vi "PendRealtime_IP5.vi"() -> ()   [LabVIEW 2012]
doc: "This VI was generated automatically using the FPGA Wizard. You can modify the VI normally."
uses:
  <vilib>/Platform/TimedLoop/XDataNode/timing_clust.ctl
  <vilib>/Platform/TimedLoop/XDataNode/nitl_modes.ctl
  <vilib>/Platform/TimedLoop/XDataNode/wakeup.ctl
  <vilib>/FPGAPlugInAG/sbRIO-9632/niLvFpga_Open_sbRIO-9632.vi
  <vilib>/rvi/interface/common/dynamic/niFpgaDynamicAddResources.vi
  <vilib>/FPGAPlugInAG/Dynamic/niLvFpga_Reset_Dynamic.vi
  <vilib>/FPGAPlugInAG/Dynamic/niLvFpga_Run_Dynamic.vi
  <vilib>/Utility/error.llb/Error Cluster From Error Code.vi
  <vilib>/rvi/errors/niLvFpgaAdjustHostInterfaceError.vi
  <vilib>/FPGAPlugInAG/Dynamic/niLvFpga_Close_Dynamic.vi
  <vilib>/rvi/interface/nirviOpenFPGA/nirviOpenFPGA.xnode
  FPGA Bitfiles/PPDControlLab3_FPGA_IP5.lvbitx
  <vilib>/rvi/interface/nirviMethod/nirviMethod.xnode
  <vilib>/Platform/TimedLoop/XDataNode/XDataNode.xnode
  <vilib>/rvi/interface/nirviReadWriteControl/nirviReadWriteControl.xnode
  <vilib>/rvi/interface/nirviCloseFPGA/nirviCloseFPGA.xnode
  SysIDRealtime.lvlib
  <vilib>/rvi/interface/Simulation/niFpgaSimulationCallBeginRW.vi
  <vilib>/Platform/TimedLoop/XDataNode/XDNodeRunTimeDep.lvlib
  NiFpgaLv.dll
panel:
  in  "K3":dbl=32.996501911713274
  in  "K4":dbl=3.4016071395471763
  in  "K1":dbl=-0.3249
  in  "K2":dbl=-1.0317
  out "Enabled":bool=TRUE
  in  "Enable Control":bool=TRUE
  out "Control":fxp<+/-,20,5>
  in  "K4'":dbl=0.002609032676032684
  in  "K3'":dbl=0.0461262
  in  "K2'":dbl=1.0317e-06
  in  "K1'":dbl=3.249e-07
  out "Pendulum Position":i32=-6910
  out "Pendulum Response":dynamicdata(graph)=[{"t0"=timestamp(0 s since 1904-01-01), "dt"=1.0, "Y"=array[8192 elements]}, {"t0"=timestamp(0 s since 1904-01-01), "dt"=1.0, "Y"=array[53587 elements]}]
  out "Ratio":fxp<+/-,32,7>
  in  "Gain":fxp<+/-,32,7>=0.006999999284744263
  in  "Radio Buttons":enum32{"Radio Selection 1", "Radio Selection 2"}(radio)
  in  "OK Button":bool
  out "Step Response":dynamicdata(graph)=[{"t0"=timestamp(0 s since 1904-01-01), "dt"=1.0, "Y"=array[8192 elements]}, {"t0"=timestamp(0 s since 1904-01-01), "dt"=1.0, "Y"=array[8192 elements]}, {"t0"=timestamp(0 s since 1904-01-01), "dt"=1.0, "Y"=array[8192 elements]}]
  in  "samples":i32=8192
  in  "Reference":i32=100000
  in  "Quad Reset":bool=TRUE
  in  "DGain":fxp<+/-,32,7>
  in  "PGain":fxp<+/-,32,7>=-0.006999999284744263
  out "Amp In":dbl[](graph)
  out "Amp Cpmmand":fxp<+/-,20,5>=-16.0
  out "Iteration Duration":i64=1663
  out "Position":i32[](graph)
  in  "Control Rate (ticks)":u32=10000
  in  "Period (us)":i64=1000
  out "Finished Late? [i-1]":bool=TRUE
  out "quad saved (Port0/DIO0,Port0/DIO1)":cluster{"Position":i32, "Index Count":u16}={"Position"=-185790, "Index Count"=8041}
  out "quad pos (Port0/DIO0,Port0/DIO1)":i32=-185792
  out "Late? Latched":bool=TRUE
  in  "Local Stop 0":bool
  in  "Start 0":bool
  in  "Loop Rate (Hz)":dbl=100000.0
  out "Calculated Rate (Hz)":dbl=100000.0
  out "error out":errorcluster
  in  "Global Stop":bool
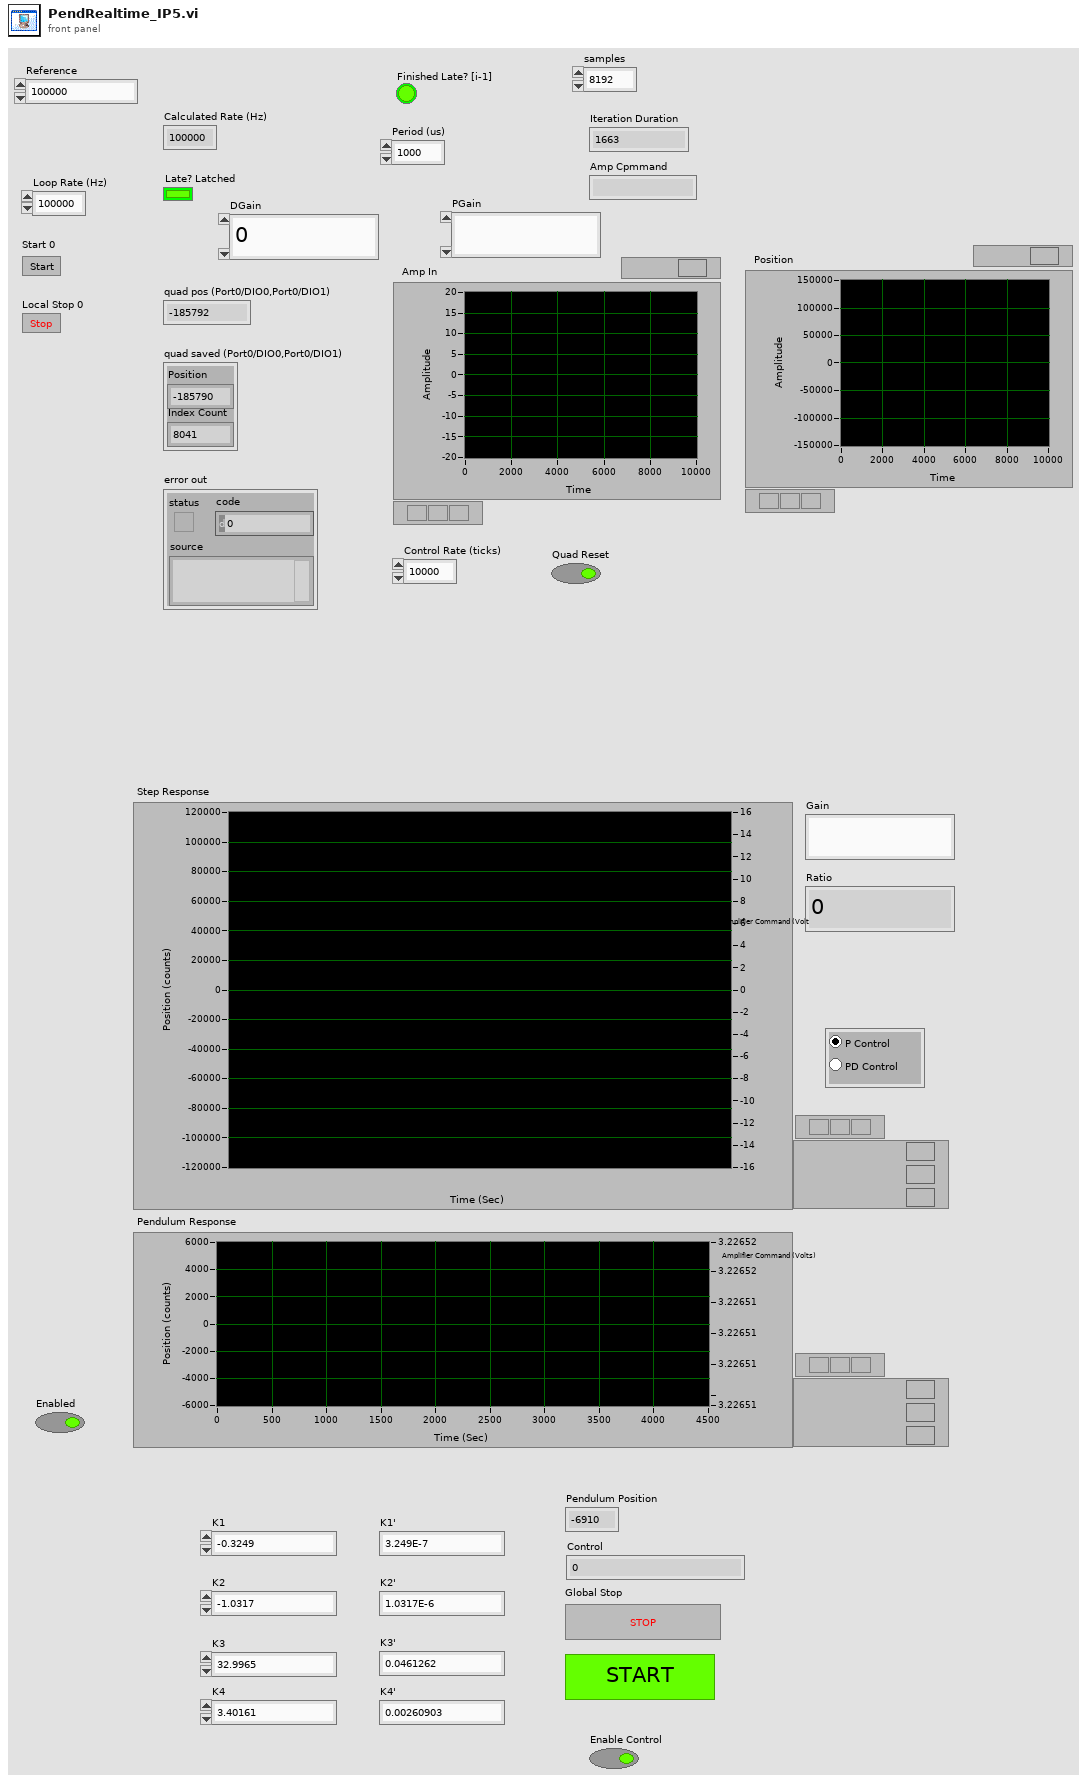
[diagram p1: front panel]
types:
  T1 = typedef "XDNodeRunTimeDep.lvlib/timing_clust.ctl" = cluster{"Expected End [f-1]":u64, "Actual End [f-1]":u64, "Finished Late? [f-1]":bool, "Expected End [i-1]":u64, "Actual End [i-1]":u64, "Finished Late? [i-1]":bool, "Expected Start [i]":u64, "Actual Start [i]":u64, "Expected Start [f]":u64, "Actual Start [f]":u64, "Source Name":string, "Structure Name":string, "Period":i64, "Deadline":i64, "Offset":i64, "Start":i64, "Priority":i32, "Timeout":i32, "Mode":T2, "Wakeup Reason":T3, "Error":errorcluster, "Source Type":string, "Secondary Source Type":string, "Global End Time":u64, "Global Start Time":u64, "Frame Duration":u64, "Iteration Duration":u64, "Assigned CPU":i32, "I/O Scan Engine Mode":u32}
  T2 = typedef "XDNodeRunTimeDep.lvlib/nitl_modes.ctl" = enum32{"No Change", "Process missed periods, maintain original phase", "Discard missed periods, maintain original phase", "Process missed periods, ignore original phase", "Discard missed periods, ignore original phase"}
  T3 = typedef "XDNodeRunTimeDep.lvlib/wakeup.ctl" = enum32{"Normal", "Aborted", "Asynchronous wakeup", "Timing source error", "Timed loop error", "Timeout"}
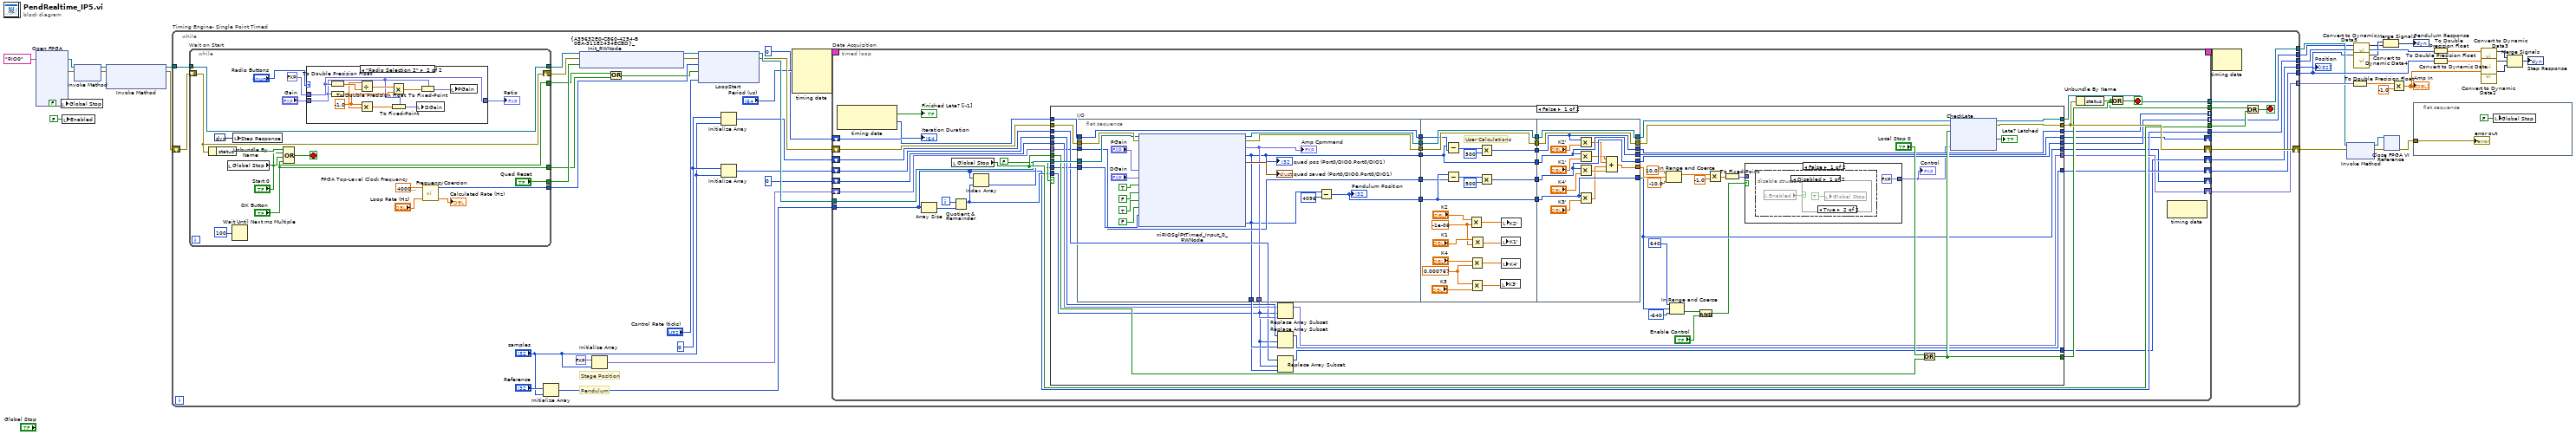
[diagram p0: block diagram]
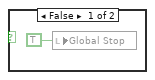
[diagram p2: hidden frame]
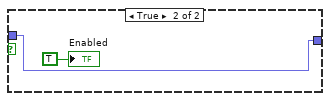
[diagram p4: hidden frame]
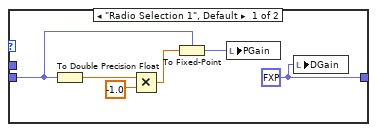
[diagram p6: hidden frame]
diagram:
  n1 = xnode ("Open FPGA")("resource name"=tag "RIO0") -> ("FPGA VI Reference Out"=w29:refnum<k20>, "error out"=w30:errorcluster)  [unwired: 1 in]
  n2 = local write "Global Stop"(FALSE ("Global Stop")) -> ()
  n3 = local write "Enabled"(FALSE ("Enabled")) -> ()
  n4 = xnode ("Invoke Method")("FPGA VI Reference In"=w29, "error in"=w30) -> ("FPGA VI Reference Out"=w12:refnum<k20>, "error out"=w11:errorcluster)
  n5 = xnode ("Invoke Method")("FPGA VI Reference In"=w12, "error in"=w11) -> ("FPGA VI Reference Out"=w17:refnum<k20>, "error out"=w31:errorcluster)  [unwired: 1 in]
  n6 = while "Timing Engine- Single Point Timed" {
    tunnel: w17 -> [w65]
    shift-right: [w64] -> w15
    shift-left: w31 -> [w68]
    tunnel: [w47] -> w23
    tunnel: [w48] -> w27
    tunnel: [w43] -> w21
    tunnel: [w39] -> w16
    tunnel: [w35] -> w7
    tunnel: [w32] -> w5
    stop <- w59 stop-if-true
    w38 = 0 ("quad pos (Port0/DIO0,Port0/DIO1)")
    # "Pendulum"
    # "Stage Position"
    n7 = while "Wait on Start" {
      tunnel: w65 -> [w240]
      tunnel: [w240] -> w63
      tunnel: [w232] -> w56
      tunnel: ["Start 0"] -> w42
      shift-right: [w234] -> w62
      shift-left: w68 -> [w234]
      tunnel: ["Quad Reset"] -> w46
      tunnel: ["OK Button"] -> w41
      stop <- w241 stop-if-true
      w235 = 40000000.0  # FPGA Top-Level Clock Frequency
      n8 = Unbundle By Name(w234) -> ("status"=w233:bool)
      n9 = local read "Global Stop"() -> (w238:bool)
      n10 = Wait Until Next ms Multiple(millisecond multiple=u32 100) -> ()  [unwired: 1 out]
      n11 = local write "Step Response"(dynamicdata [] ("Step Response")) -> ()
      n12 = Compound Arithmetic op=OR(w233, "Start 0", w238, "OK Button") -> (w241:bool)
      n13 = case shown="\"Radio Selection 2\"" "Radio Buttons" {
        tunnel: "Gain" -> [w243 w249]
        tunnel: fxp<+/-,32,7> 40.0 ("Ratio") -> [_ w254]
        tunnel: [w247 w254] -> w225
        frame "Radio Selection 1", Default {
          w247 = fxp<+/-,32,7> 0.0 ("DGain")
          n14 = To Double Precision Float(number=w243) -> (double precision float=w246:dbl)
          n15 = Multiply(x=w246, y=-1.0) -> (x*y=w244:dbl)
          n16 = To Fixed-Point(fixed-point type=w243, number=w244) -> (fixed-point=w242:fxp<+/-,32,7>)
          n17 = local write "PGain"(w242) -> ()
          n18 = local write "DGain"(w247) -> ()
        }
        frame "Radio Selection 2" {
          w252 = -1.0 ("y")
          n19 = To Double Precision Float(number=w254) -> (double precision float=w257:dbl)
          n20 = To Double Precision Float(number=w249) -> (double precision float=w251:dbl)
          n21 = Divide(x=w251, y=w257) -> (x/y=w256:dbl)
          n22 = Multiply(x=w252, y=w251) -> (x*y=w250:dbl)
          n23 = Multiply(x=w256, y=w252) -> (x*y=w253:dbl)
          n24 = To Fixed-Point(fixed-point type=w249, number=w250) -> (fixed-point=w248:fxp<+/-,32,7>)
          n25 = local write "DGain"(w248) -> ()
          n26 = To Fixed-Point(fixed-point type=w249, number=w253) -> (fixed-point=w255:fxp<+/-,32,7>)
          n27 = local write "PGain"(w255) -> ()
        }
      }
      "Ratio" <- w225
      n28 = call "FrequencyCoercion.vi"("Loop Rate (Hz)"="Loop Rate (Hz)", "FPGA Top-Level Clock Frequency"=w235) -> ("Actual Rate (Hz)"=→"Calculated Rate (Hz)":dbl, "FPGA Ticks"=w232:u32)  [unwired: 2 in]
    }
    n29 = Initialize Array("Reference", "samples") -> (w44:i32[])
    n30 = xnode ("{A39632E0-C860-4254-B0EA-311E2434ECBD}_Init_RWNode")("FPGA VI Reference In"=w63, "error in"=w62, "quad reset (Port0/DIO0,Port0/DIO1)"=w46) -> ("FPGA VI Reference Out"=w57:refnum<k20>, "error out"=w61:errorcluster)
    n31 = Initialize Array(fxp<+/-,20,5> 0.0 ("Amp Cpmmand"), "samples") -> (w49:fxp<+/-,20,5>[])
    n32 = Or(x=w42, y=w41) -> (x .or. y?=w40:bool)
    n33 = xnode ("LoopStart")("FPGA VI Reference In"=w57, "error in"=w61, "Loop Rate (Ticks)"=w56, "Start 0"=w40, "Control Rate (ticks)"="Control Rate (ticks)") -> ("FPGA VI Reference Out"=w67:refnum<k20>, "error out"=w66:errorcluster)
    n34 = Initialize Array(w38, "samples") -> (w36:i32[])
    n35 = Initialize Array(w38, "samples") -> (w51:i32[])
    n36 = node-c288("Period (us)") -> (w55:T1)  [unwired: 3 in]
    n37 = timed-loop "Data Acquisition" {
      tunnel: w67 -> [w91]
      tunnel: [w93] -> w60
      tunnel: [w92] -> w58
      shift-right: [w96] -> w64
      shift-left: w66 -> [w90]
      timing: w55 -> [_]
      timing-out: [_] -> w54
      tunnel: w44 -> [w78]
      shift-right: [w79] -> w48
      shift-left: w49 -> [w81]
      shift-right: [w80] -> w47
      shift-left: w51 -> [w83]
      tunnel: [w78] -> w43
      tunnel: [w77] -> w39
      shift-right: [w75] -> w35
      shift-left: w36 -> [w76]
      shift-right: [w72] -> _
      shift-left: 0 ("Pendulum Position") -> [w74]
      shift-right: [w70] -> _
      shift-left: 0 ("Stage Position") -> [w73]
      tunnel: [w69] -> _ mode=indexing
      tunnel: [w71] -> w32 mode=indexing
      i -> [w87]
      stop <- w94 stop-if-true
      n38 = node-c288() -> (→"Finished Late? [i-1]":bool, →"Iteration Duration":i64)  [unwired: 1 in]
      n39 = Array Size(array=w78) -> (size(s)=w85:i32)
      n40 = local read "Global Stop"() -> (w93:bool)
      n41 = Quotient & Remainder(x=w87, y=w85) -> (x-y*floor(x/y)=w84:i32)  [unwired: 1 out]
      n42 = Index Array(array=w78, index=w84) -> (element=w86:i32)
      n43 = case "Timeout" shown="False" FALSE {
        tunnel: w91 -> [w147 w217]
        tunnel: w90 -> [w146 w219]
        tunnel: [w140 w219] -> w96
        tunnel: [w142 w218] -> w95
        tunnel: w93 -> [w143 w218]
        tunnel: w86 -> [w133 _]
        tunnel: w84 -> [w130 _]
        tunnel: w83 -> [w138 _]
        tunnel: [w137 _] -> w80
        tunnel: w81 -> [w136 _]
        tunnel: [w134 _] -> w79
        tunnel: [w132 w217] -> w77
        tunnel: w76 -> [w131 _]
        tunnel: [w128 _] -> w75
        tunnel: [w110 w215] -> w72
        tunnel: [w125 w216] -> w70
        tunnel: w74 -> [w121 w215]
        tunnel: w73 -> [w119 w216]
        tunnel: [w118 _] -> w71
        tunnel: [w116 _] -> w69
        frame False {
          n44 = flat-sequence "I/O" {
            tunnel: w147 -> [w175]
            tunnel: w146 -> [w177]
            tunnel: [w176] -> w152
            tunnel: [w174] -> w149
            tunnel: [w162] -> w139
            tunnel: [w172] -> w135
            tunnel: w133 -> [w165]
            tunnel: [w161] -> w129
            tunnel: [w159] -> w126
            tunnel: [w162] -> w123
            tunnel: [w164] -> w122
            tunnel: w121 -> [w164]
            tunnel: [w163] -> w120
            tunnel: w119 -> [w163]
            tunnel: [w199] -> w151
            tunnel: w152 -> [w198]
            tunnel: w149 -> [w199]
            tunnel: [w198] -> w150
            tunnel: [w197] -> w127
            tunnel: w126 -> [w197]
            tunnel: [w194] -> w124
            tunnel: w123 -> [w194]
            tunnel: w122 -> [w196]
            tunnel: w120 -> [w195]
            tunnel: [w191] -> w117
            tunnel: [w188] -> w115
            tunnel: [w213] -> w145
            tunnel: [w214] -> w148
            tunnel: w151 -> [w214]
            tunnel: w150 -> [w213]
            tunnel: [w207] -> w110
            tunnel: w127 -> [w207]
            tunnel: [w205] -> w125
            tunnel: w124 -> [w205]
            tunnel: [w208] -> w118
            tunnel: w117 -> [w208]
            tunnel: [w206] -> w116
            tunnel: w115 -> [w206]
            tunnel: [w200] -> w114
            frame #0 {
              n45 = xnode ("niRIOSglPtTimed_Input_0_RWNode")("FPGA VI Reference In"=w175, "error in"=w177, "PGain"="PGain", "DGain"="DGain", "Amp Enable"=TRUE, "Amp Reset"=FALSE, "Brake"=TRUE, "quad reset (Port0/DIO0,Port0/DIO1)"=FALSE, "Reference"=w165) -> ("FPGA VI Reference Out"=w174:refnum<k20>, "error out"=w176:errorcluster, "Amp Cpmmand"=w172:fxp<+/-,20,5>, "Stage Position"=w162:i32, "quad saved (Port0/DIO0,Port0/DIO1)"=→"quad saved (Port0/DIO0,Port0/DIO1)":cluster{"Position":i32, "Index Count":u16}, "Pendulum Position"=w161:i32)
              "quad pos (Port0/DIO0,Port0/DIO1)" <- w162
              "Amp Cpmmand" <- w172
              n46 = Subtract(x=w161, y=4096 ("x")) -> (x-y=w159:i32)
              "Pendulum Position" <- w159
            }
            frame #1 {
              w179 = 0.000767 ("y")
              w184 = -1e-06 ("y")
              # "User Calculations"
              n47 = Subtract(x=w194, y=w195) -> (x-y=w190:i32)
              n48 = Subtract(x=w197, y=w196) -> (x-y=w193:i32)
              n49 = Multiply(x="K2", y=w184) -> (x*y=w186:dbl)
              n50 = Multiply(x="K4", y=w179) -> (x*y=w181:dbl)
              n51 = Multiply(x=w179, y="K3") -> (x*y=w178:dbl)
              n52 = Multiply(x="K1", y=w184) -> (x*y=w183:dbl)
              n53 = Multiply(x=w190, y=500) -> (x*y=w188:i32)
              n54 = Multiply(x=w193, y=500) -> (x*y=w191:i32)
              n55 = local write "K3'"(w178) -> ()
              n56 = local write "K1'"(w183) -> ()
              n57 = local write "K4'"(w181) -> ()
              n58 = local write "K2'"(w186) -> ()
            }
            frame #2 {
              n59 = Multiply(x=w206, y="K2'") -> (x*y=w202:dbl)
              n60 = Multiply(x=w205, y="K1'") -> (x*y=w201:dbl)
              n61 = Multiply(x=w208, y="K4'") -> (x*y=w204:dbl)
              n62 = Multiply(x=w207, y="K3'") -> (x*y=w203:dbl)
              n63 = Compound Arithmetic op=ADD(w201, w202, w203, w204) -> (w200:dbl)
            }
          }
          n64 = Replace Array Subset(array=w136, new element=w135, index=w130) -> (w134:fxp<+/-,20,5>[])
          n65 = Replace Array Subset(array=w138, new element=w139, index=w130) -> (w137:i32[])
          n66 = Replace Array Subset(array=w131, new element=w129, index=w130) -> (w128:i32[])
          n67 = In Range and Coerce(upper limit=10.0, x=w114, lower limit=-10.0) -> (coerced(x)=w111:dbl)  [unwired: 1 out]
          n68 = In Range and Coerce(upper limit=640, x=w110, lower limit=-640) -> (In Range?=w105:bool)  [unwired: 1 out]
          n69 = And(x=w105, y="Enable Control") -> (x .and. y?=w104:bool)
          n70 = Multiply(x=w111, y=-1.0) -> (x*y=w102:dbl)
          n71 = To Fixed-Point(number=w102) -> (fixed-point=w107:fxp<+/-,20,5>)  [unwired: 1 in]
          n72 = case shown="False" w104 {
            tunnel: w107 -> [_ w158]
            tunnel: [fxp<+/-,20,5> 0.0 w158] -> w106
            frame False {
              n73 = disable-structure shown="Disabled" {
                frame Disabled {
                  n74 = local read "Enabled"() -> (w154:bool)
                  n75 = case shown="True" w154 {
                    frame False {
                      n76 = local write "Global Stop"(TRUE ("Global Stop")) -> ()
                    }
                    frame True {
                      n77 = local write "Global Stop"(TRUE ("Global Stop")) -> ()
                    }
                  }
                }
                frame Enabled {
                }
              }
            }
            frame True {
              "Enabled" <- TRUE ("Enabled")
            }
          }
          "Control" <- w106
          n78 = Or(x="Local Stop 0", y=w143) -> (x .or. y?=w142:bool)
          n79 = xnode ("CheckLate")("FPGA VI Reference In"=w148, "error in"=w145, "Local Stop 0"=w142, "State_Control"=w106) -> ("FPGA VI Reference Out"=w132:refnum<k20>, "error out"=w140:errorcluster, "Late? Latched"=→"Late? Latched":bool)
        }
        frame True {
          # "Timeout waiting for an interrupt. This case checks the state of the global stop.\nIf global stop is not set, then loop around to wait for an interrupt again."
        }
      }
      n80 = Unbundle By Name(w96) -> ("status"=w92:bool)
      n81 = Or(x=w92, y=w95) -> (x .or. y?=w94:bool)
      n82 = node-c288() -> ()  [unwired: 1 in, 1 out]
    }
    n83 = node-c288(w54) -> ()  [unwired: 1 out]
    n84 = Or(x=w58, y=w60) -> (x .or. y?=w59:bool)
  }
  "Position" <- w23
  n85 = xnode "Invoke Method"("FPGA VI Reference In"=w16, "error in"=w15) -> ("FPGA VI Reference Out"=w14:refnum<k20>, "error out"=w13:errorcluster)
  n86 = To Double Precision Float(number=w27) -> (double precision float=w9:dbl[])
  n87 = call "Convert to Dynamic Data5"("Array"=w5) -> ("Dynamic Data Type"=w4:dynamicdata)  [unwired: 3 in]
  n88 = call "Convert to Dynamic Data4"("Array"=w7) -> ("Dynamic Data Type"=w6:dynamicdata)  [unwired: 3 in]
  n89 = Merge Signals(w6, w4) -> (→"Pendulum Response":dynamicdata)
  n90 = xnode ("Close FPGA VI Reference")("FPGA VI Reference In"=w14, "error in"=w13) -> ("error out"=w28:errorcluster)
  n91 = Multiply(x=w9, y=-1.0) -> (x*y=w8:dbl[])
  "Amp In" <- w8
  n92 = flat-sequence {
    tunnel: w28 -> [w259]
    frame #0 {
      n93 = local write "Global Stop"(FALSE ("Global Stop")) -> ()
      "error out" <- w259
    }
  }
  n94 = To Double Precision Float(number=w21) -> (double precision float=w20:dbl[])
  n95 = To Double Precision Float(number=w23) -> (double precision float=w22:dbl[])
  n96 = call "Convert to Dynamic Data3"("Array"=w20) -> ("Dynamic Data Type"=w19:dynamicdata)  [unwired: 3 in]
  n97 = call "Convert to Dynamic Data"("Array"=w22) -> ("Dynamic Data Type"=w25:dynamicdata)  [unwired: 3 in]
  n98 = call "Convert to Dynamic Data2"("Array"=w8) -> ("Dynamic Data Type"=w24:dynamicdata)  [unwired: 3 in]
  n99 = Merge Signals(w19, w25, w24) -> (→"Step Response":dynamicdata)
